vi "dfd_FXP PtByPt Lattice Allpass (one multiplier).vi"(6 "state in":i64[](array[numeric]), 7 "FXPOPs":T5[](array[typedef]) {"source" items=["Coef a/k"=0, "Coef b/v"=7, "Input"=1, "Output"=2, "Multiplicand"=3, "Product"=4, "Sum"=5, "Delay"=6, "Gain"=8]}, 8 "filtering statistics in":T4(array[cluster]) {"statistics information"."min value" format="%.2f"; "statistics information"."max value" format="%.2f"; "Quantizer Source" items=["Coefficients a/k"=0, "Coefficients b/v"=7, "Input"=1, "Output"=2, "Multiplicand"=3, "Product"=4, "Sum"=5, "Delay"=6]}, 10 "coef k[M..1]":T1, 11 "x":T7={"value"=0, "wl"=0, "iwl"=0, "Signed"=TRUE} {"value" format="%.0x"}) -> (0 "filtering statistics out":T4(array[cluster]) {"statistics information"."min value" format="%.2f"; "statistics information"."max value" format="%.2f"; "Quantizer Source" items=["Coefficients a/k"=0, "Coefficients b/v"=7, "Input"=1, "Output"=2, "Multiplicand"=3, "Product"=4, "Sum"=5, "Delay"=6]}, 3 "filtered x":T7={"value"=0, "wl"=0, "iwl"=0, "Signed"=TRUE} {"value" format="%.0x"}, 4 "state out":i64[](array[numeric]))   [LabVIEW 2017, in "NI_DigFilter_FXP.lvlib"]
uses:
  <vilib>/addons/Digital Filter Design/NI_DigFilter_FXP.lvlib
  <vilib>/addons/Digital Filter Design/_Objects.llb/dfd_DFXP Data Type (scaler).ctl
  <vilib>/addons/Digital Filter Design/_Objects.llb/dfd_DFXP Operation Parameter.ctl
  <vilib>/addons/Digital Filter Design/_Objects.llb/dfd_Internal Quantization Srcs.ctl
  <vilib>/addons/Digital Filter Design/_Objects.llb/dfd_DFXP Data Type (vector).ctl
  <vilib>/addons/Digital Filter Design/_Objects.llb/DFD Quantization Sources.ctl
  <vilib>/addons/Digital Filter Design/_Objects.llb/DFD FXP Statistics Data.ctl
  <vilib>/addons/Digital Filter Design/NI_DigFilterLicensed.lvlib
panel:
  in  "DFXP array type":T1
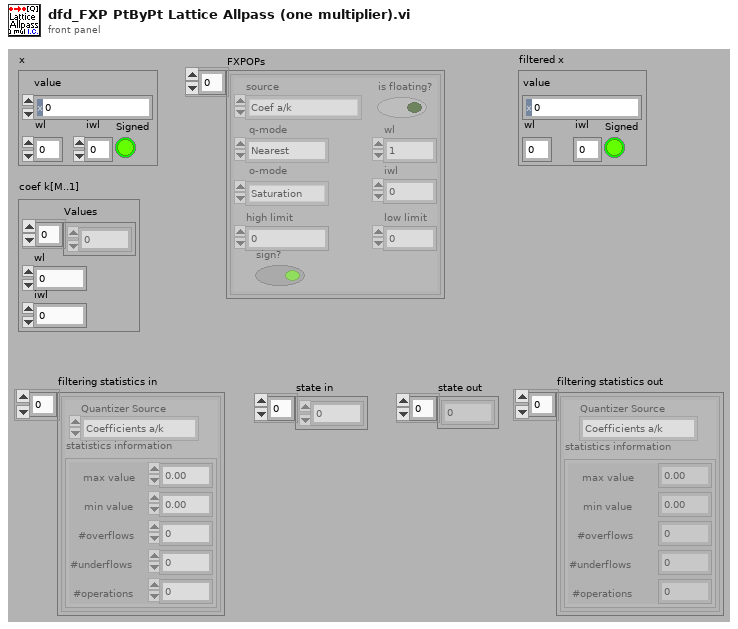
[diagram p1: front panel]
types:
  T1 = typedef "dfd_DFXP Data Type (vector).ctl" = cluster{"Values":i64[], "wl":i16, "iwl":i16}
  T2 = typedef "NI_DigFilterLicensed.lvlib/DFD Quantization Sources.ctl" = u16
  T3 = typedef "NI_DigFilterLicensed.lvlib/DFD FXP Statistics Data.ctl" = cluster{"max value":ext, "min value":ext, "#overflows":i32, "#underflows":i32, "#operations":i32}
  T4 = cluster{"Quantizer Source":T2, "statistics information":T3}[]
  T5 = typedef "dfd_DFXP Operation Parameter.ctl" = cluster{"source":T6, "is floating?":bool, "o-mode":enum16{"Saturation", "Wrap"}, "q-mode":enum16{"Nearest", "Truncation"}, "wl":i16, "high limit":i64, "low limit":i64, "iwl":i16, "sign?":bool}
  T6 = typedef "NI_DigFilterLicensed.lvlib/dfd_Internal Quantization Srcs.ctl" = u16
  T7 = typedef "dfd_DFXP Data Type (scaler).ctl" = cluster{"value":i64, "wl":i16, "iwl":i16, "Signed":bool}
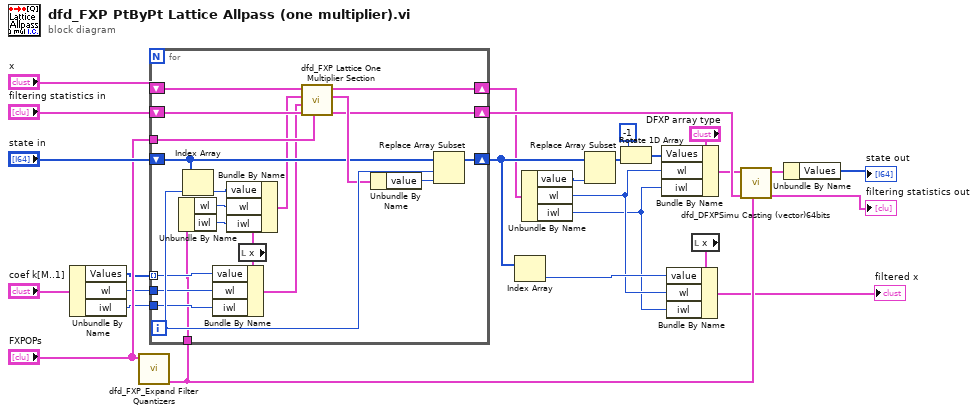
[diagram p0: block diagram]
diagram:
  n1 = Unbundle By Name("coef k[M..1]") -> ("Values"=w13:i64[], "wl"=w12:i16, "iwl"=w11:i16)
  n2 = call <vilib>:"dfd_FXP_Expand Filter Quantizers.vi"("FXPOPs"="FXPOPs") -> ("Delay"=w10:T5)  [unwired: 10 out]
  n3 = for {
    shift-right: [w43] -> w9
    shift-left: "x" -> [w45]
    shift-right: [w46] -> w22
    shift-left: "state in" -> [w37]
    tunnel: "FXPOPs" -> [w42]
    shift-right: [w39] -> w21
    shift-left: "filtering statistics in" -> [w41]
    tunnel: w13 -> [w36] mode=indexing
    tunnel: w12 -> [w34]
    tunnel: w11 -> [w33]
    tunnel: w10 -> [w30]
    i -> [w44]
    n4 = Unbundle By Name(w30) -> ("wl"=w29:i16, "iwl"=w28:i16)
    n5 = Index Array(array=w37, index=w44) -> (element=w38:i64)
    n6 = local read "x"() -> (w31:T7)
    n7 = Bundle By Name(cluster=w31, "value"=w36, "wl"=w34, "iwl"=w33) -> (w35:T7)
    n8 = Bundle By Name(cluster=w31, "value"=w38, "wl"=w29, "iwl"=w28) -> (w32:T7)
    n9 = call <vilib>:"dfd_FXP Lattice One Multiplier Section.vi"("FXPOPs"=w42, "filtering statistics in"=w41, "k(m)"=w35, "w(m-1)"=w32, "x(m)"=w45) -> ("filtering statistics out"=w39:T4, "w(m)"=w40:T7, "x(m-1)"=w43:T7)  [unwired: 1 out]
    n10 = Unbundle By Name(w40) -> ("value"=w27:i64)
    n11 = Replace Array Subset(array=w37, new element=w27, index=w44) -> (w46:i64[])
  }
  n12 = Index Array(array=w22) -> (element=w20:i64)  [unwired: 1 in]
  n13 = Unbundle By Name(w9) -> ("value"=w8:i64, "wl"=w3:i16, "iwl"=w2:i16)
  n14 = Replace Array Subset(array=w22, new element=w8) -> (w24:i64[])  [unwired: 1 in]
  n15 = Rotate 1D Array(1:w24, 2:-1 ("n")) -> (0:w16:i64[])
  n16 = Bundle By Name(cluster="DFXP array type", "Values"=w16, "wl"=w3, "iwl"=w2) -> (w7:T1)
  n17 = local read "x"() -> (w4:T7)
  n18 = Bundle By Name(cluster=w4, "value"=w20, "wl"=w3, "iwl"=w2) -> (→"filtered x":T7)
  n19 = call <vilib>:"dfd_DFXPSimu Casting (vector)64bits.vi"("op params"=w10, "filtering statistics in"=w21, "Value in"=w7) -> ("filtering statistics out"=→"filtering statistics out":T4, "Value out"=w15:T1)  [unwired: 1 in, 6 out]
  n20 = Unbundle By Name(w15) -> ("Values"=→"state out":i64[])
